vi "All Child Values.vi"(11 "Entity in":refnum<class "Entity.lvclass">) -> (2 "All Values":refnum<class "Type.lvclass">[](array[class]))   [LabVIEW 2020, in "Conditum.lvlib" / "Entity.lvclass"]
uses:
  Entity.lvclass
  Columns/Type/Type.lvclass
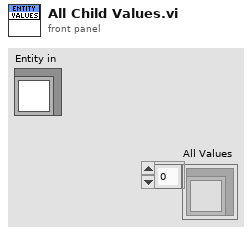
[diagram p1: front panel]
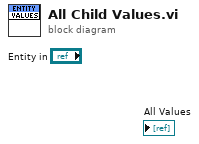
[diagram p0: block diagram]
diagram:
